vi "Clear.vi"(8 "error in (no error)":errorcluster, 11 "Mock Process In":refnum<class "Mock Error Handler.lvclass">) -> (0 "error out":errorcluster)   [LabVIEW 2020, in "Mock Error Handler.lvclass"]
doc: "Clears any resorces allocated during initialization."
uses:
  Mock Error Handler.lvclass
  Mock Error Handler.lvclass/Mock Error Handler.ctl
  Framework/Base/Base.lvclass
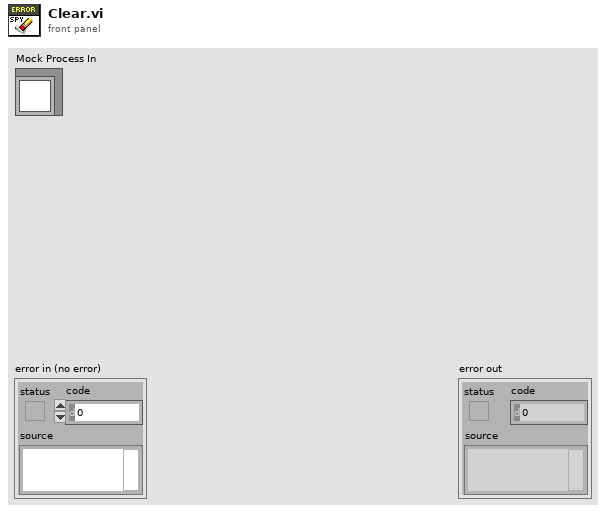
[diagram p1: front panel]
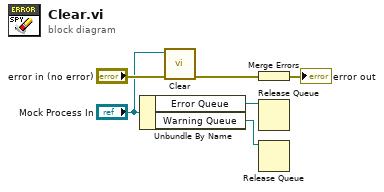
[diagram p0: block diagram]
diagram:
  n1 = Unbundle By Name("Mock Process In") -> ("Error Queue"=w4:refnum<queue>, "Warning Queue"=w1:refnum<queue>)
  n2 = call-parent "Clear.vi"("error in (no error)"="error in (no error)", "Base In"="Mock Process In") -> ("error out"=w3:errorcluster)  [unwired: 9 in]
  n3 = Merge Errors(w3) -> (→"error out":errorcluster)
  n4 = Release Queue(queue=w4) -> ()  [unwired: 2 in, 3 out]
  n5 = Release Queue(queue=w1) -> ()  [unwired: 2 in, 3 out]
